vi "SimpleOut.vi"() -> ()   [LabVIEW 2020]
uses:
  <vilib>/measure/NI_MABase.lvlib
panel:
  in  "stop (F)":bool
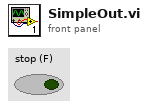
[diagram p1: front panel]
types:
  T1 = enum16{"Sine Wave", "Triangle Wave", "Square Wave", "Sawtooth Wave"}
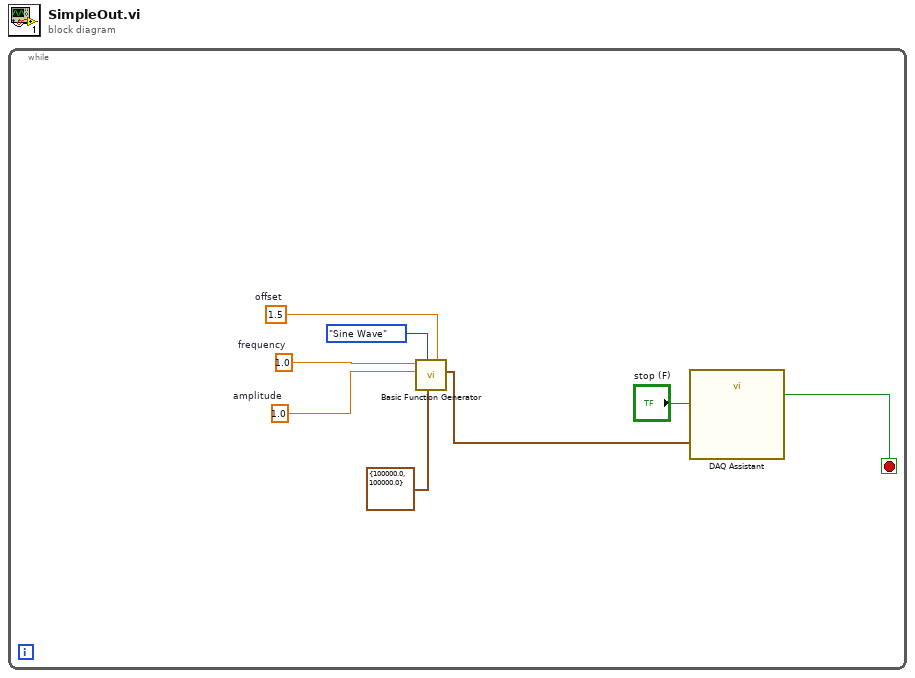
[diagram p0: block diagram]
diagram:
  n1 = while {
    stop <- w7 stop-if-true
    w2 = 1.5  # offset
    w3 = 1.0  # frequency
    w4 = 1.0  # amplitude
    n2 = call <vilib>:"Basic Function Generator.vi"("offset"=w2, "sampling info"=cluster{"Fs":dbl, "#s":dbl} {"Fs"=100000.0, "#s"=100000.0}, "signal type"=T1."Sine Wave", "amplitude"=w4, "frequency"=w3) -> ("signal out"=w6:waveform(dbl))  [unwired: 4 in, 2 out]
    n3 = call "DAQ Assistant"("data"=w6, "stop (F)"="stop (F)") -> ("stopped"=w7:bool)  [unwired: 15 in, 2 out]
  }
